vi "SIM Simulation init.vi"(0 "initial time":dbl format="%.2f", 1 "Nan/Inf Check":bool, 2 "continuous integrator":T3, 3 "Execution Mode":T1 items=["Simulate to Completion", "Single Time-Step Simulation (Fixed Step Only)"], 5 "final time":dbl=10.0 format="%.2f", 7 "time step":dbl=0.1 format="%.2f", 8 "error in (no error)":errorcluster, 9 "absolute tolerance":dbl=0.1 format="%.2e", 11 "relative tolerance":dbl=0.1 format="%.2e", 12 "maximum step size":dbl=0.1 format="%.2e", 13 "min step size":dbl=0.1, 14 "discrete time step":dbl=0.1, 15 "Simulation data":T2={"continuous integrator"=enum."RK 1 (Euler)", "initial time"=0.0, "final time"=0.0, "step size"=0.0, "proposed step size"=0.0, "max step size"=0.0, "min step size"=0.0, "discrete time step"=0.0, "max step ratio"=0.0, "Diag Eval Stage"=enum."Init", "Substep Index"=0, "Timestep Index"=0.0, "simulation time"=0.0, "current timestep base"=0.0, "proposed step time"=0.0, "absolute tolerance"=0.0, "relative tolerance"=0.0, "step accepted?"=TRUE, "step complete?"=FALSE, "Halt?"=FALSE, "reset integrator?"=FALSE, "machine epsilon"=0.0, "min float"=0.0, "error"={"status"=FALSE, "code"=0, "source"=""}, "Method Order"=0, "Finished Late [i-1]"=FALSE, "Discrete step?"=FALSE, "NaN and Inf check?"=FALSE, "Final Timestep Index"=0.0, "(maj+disc)or(init)?"=FALSE, "Full Solver Reset"=TRUE, "Execution Mode"=0, "check vector sizes?"=TRUE, "solver handles zc?"=FALSE, "Simulation Registry"={"Current Idx"=0, "Node Tags"=[], "Node Headers"=[], "Node Data"=[], "Cont State data"={"inputs"=[], "outputs"=[], "reset"=[], "lower limits"=[], "upper limits"=[], "limit types"=[], "reset types"=[], "initial conditions"=[], "reset I.C."=[], "limited?"=[], "State Names"=[]}, "DiscreteInfo"={"tick period (sec)"=0.0, "time (ticks)"=0, "fire?"=[], "registry"={"period (sec)"=[], "skew (sec)"=[], "period (tick)"=[], "skew (tick)"=[]}, "discrete \nblocks?"=FALSE, "steps per tick"=0.0, "steps to tick"=0.0, "discrete \ntick?"=FALSE}, "Disc State data"={"Disc States"=[], "State Names"=[]}, "Registry Error"={"Error Block ID"=0, "code"=0}, "ZC Indices"=[]}, "variable step solver?"=FALSE, "First Substep?"=FALSE, "Continuous States?"=FALSE} {"Execution Mode" items=["Simulate to Completion", "Single Time-Step Simulation (Fixed Step Only)"]; "min float" format="%.1e"; "proposed step size" format="%.1e"; "proposed step time" format="%.1e"; "max step ratio" format="%.1e"; "min step size" format="%.1e"; "machine epsilon" format="%.1e"; "discrete time step" format="%.1e"; "max step size" format="%.1e"; "current timestep base" format="%.1e"; "final time" format="%.1e"; "simulation time" format="%.1e"; "relative tolerance" format="%.1e"; "absolute tolerance" format="%.1e"; "Substep Index" format="%.1e"; "step size" format="%.1e"; "initial time" format="%.1e"}) -> (10 "Simulation data out":T2={"continuous integrator"=enum."RK 1 (Euler)", "initial time"=0.0, "final time"=0.0, "step size"=0.0, "proposed step size"=0.0, "max step size"=0.0, "min step size"=0.0, "discrete time step"=0.0, "max step ratio"=0.0, "Diag Eval Stage"=enum."Init", "Substep Index"=0, "Timestep Index"=0.0, "simulation time"=0.0, "current timestep base"=0.0, "proposed step time"=0.0, "absolute tolerance"=0.0, "relative tolerance"=0.0, "step accepted?"=TRUE, "step complete?"=FALSE, "Halt?"=FALSE, "reset integrator?"=FALSE, "machine epsilon"=0.0, "min float"=0.0, "error"={"status"=FALSE, "code"=0, "source"=""}, "Method Order"=0, "Finished Late [i-1]"=FALSE, "Discrete step?"=FALSE, "NaN and Inf check?"=FALSE, "Final Timestep Index"=0.0, "(maj+disc)or(init)?"=FALSE, "Full Solver Reset"=TRUE, "Execution Mode"=0, "check vector sizes?"=TRUE, "solver handles zc?"=FALSE, "Simulation Registry"={"Current Idx"=0, "Node Tags"=[], "Node Headers"=[], "Node Data"=[], "Cont State data"={"inputs"=[], "outputs"=[], "reset"=[], "lower limits"=[], "upper limits"=[], "limit types"=[], "reset types"=[], "initial conditions"=[], "reset I.C."=[], "limited?"=[], "State Names"=[]}, "DiscreteInfo"={"tick period (sec)"=0.0, "time (ticks)"=0, "fire?"=[], "registry"={"period (sec)"=[], "skew (sec)"=[], "period (tick)"=[], "skew (tick)"=[]}, "discrete \nblocks?"=FALSE, "steps per tick"=0.0, "steps to tick"=0.0, "discrete \ntick?"=FALSE}, "Disc State data"={"Disc States"=[], "State Names"=[]}, "Registry Error"={"Error Block ID"=0, "code"=0}, "ZC Indices"=[]}, "variable step solver?"=FALSE, "First Substep?"=FALSE, "Continuous States?"=FALSE} {"Execution Mode" items=["Simulate to Completion", "Single Time-Step Simulation (Fixed Step Only)"]; "min float" format="%.1e"; "proposed step size" format="%.1e"; "proposed step time" format="%.1e"; "max step ratio" format="%.1e"; "min step size" format="%.1e"; "machine epsilon" format="%.1e"; "discrete time step" format="%.1e"; "max step size" format="%.1e"; "current timestep base" format="%.1e"; "final time" format="%.1e"; "simulation time" format="%.1e"; "relative tolerance" format="%.1e"; "absolute tolerance" format="%.1e"; "Substep Index" format="%.1e"; "step size" format="%.1e"; "initial time" format="%.1e"})   [LabVIEW 2010]
uses:
  SIM simulation data.ctl
  SIM integration method.ctl
  SIM diagram eval stage.ctl
  SIMSCR Execution Mode.ctl
  SIM Simulation Registry.ctl
  SIM Registry Node Header.ctl
  SIM Registry Node Record.ctl
  SIM trigger type.ctl
  SIM solver state data.ctl
  SIM limit type.ctl
  SIM discrete data.ctl
  SIM Discrete state data.ctl
  SIM Simulation Registry Error.ctl
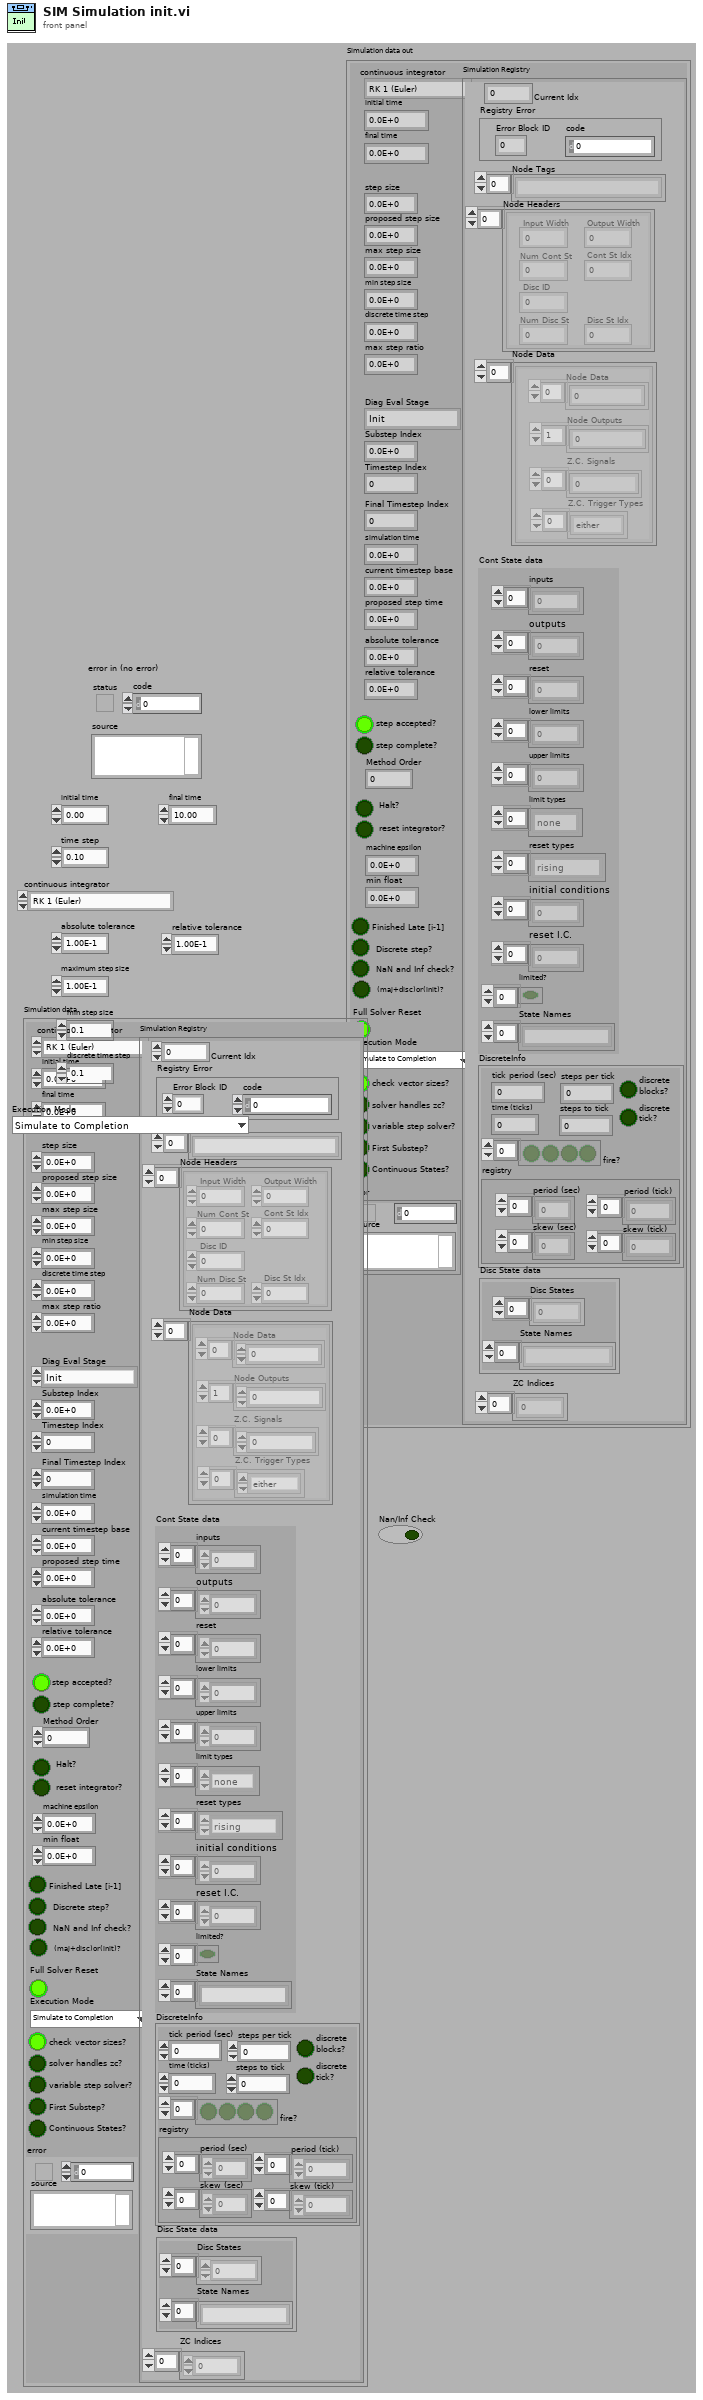
[diagram p1: front panel]
types:
  T1 = typedef "SIMSCR Execution Mode.ctl" = u16
  T2 = typedef "SIM simulation data.ctl" = cluster{"continuous integrator":T3, "initial time":dbl, "final time":dbl, "step size":dbl, "proposed step size":dbl, "max step size":dbl, "min step size":dbl, "discrete time step":dbl, "max step ratio":dbl, "Diag Eval Stage":T4, "Substep Index":i32, "Timestep Index":dbl, "simulation time":dbl, "current timestep base":dbl, "proposed step time":dbl, "absolute tolerance":dbl, "relative tolerance":dbl, "step accepted?":bool, "step complete?":bool, "Halt?":bool, "reset integrator?":bool, "machine epsilon":dbl, "min float":dbl, "error":errorcluster, "Method Order":u32, "Finished Late [i-1]":bool, "Discrete step?":bool, "NaN and Inf check?":bool, "Final Timestep Index":dbl, "(maj+disc)or(init)?":bool, "Full Solver Reset":bool, "Execution Mode":T1, "check vector sizes?":bool, "solver handles zc?":bool, "Simulation Registry":T5, "variable step solver?":bool, "First Substep?":bool, "Continuous States?":bool}
  T3 = typedef "SIM integration method.ctl" = enum16{"RK 1 (Euler)", "Linearizer", "State Query", "Trim Eval", "Adams", "RK 3", "RK 4", "RK 45", "BDF", "RK 2", "RK 23", "Rosenbrock", "Discrete States Only"}
  T4 = typedef "SIM diagram eval stage.ctl" = enum16{"Init", "Minor Substep", "Major Substep", "Final"}
  T5 = typedef "SIM Simulation Registry.ctl" = cluster{"Current Idx":i32, "Node Tags":string[], "Node Headers":T6[], "Node Data":T7[], "Cont State data":T9, "DiscreteInfo":T11, "Disc State data":T12, "Registry Error":T13, "ZC Indices":i32[]}
  T6 = typedef "SIM Registry Node Header.ctl" = cluster{"Input Width":i32, "Disc ID":i32, "Num Cont St":i32, "Cont St Idx":i32, "Num Disc St":i32, "Disc St Idx":i32, "Output Width":i32}
  T7 = typedef "SIM Registry Node Record.ctl" = cluster{"Node Data":dbl[], "Node Outputs":dbl[], "Z.C. Signals":dbl[], "Z.C. Trigger Types":T8[]}
  T8 = typedef "SIM trigger type.ctl" = enum16{"rising", "falling", "either", "none"}
  T9 = typedef "SIM solver state data.ctl" = cluster{"inputs":dbl[], "outputs":dbl[], "reset":dbl[], "lower limits":dbl[], "upper limits":dbl[], "limit types":T10[], "reset types":T8[], "initial conditions":dbl[], "reset I.C.":dbl[], "limited?":bool[], "State Names":string[]}
  T10 = typedef "SIM limit type.ctl" = enum16{"upper", "lower", "both", "none"}
  T11 = typedef "SIM discrete data.ctl" = cluster{"tick period (sec)":dbl, "time (ticks)":i32, "fire?":bool[], "registry":cluster{"period (sec)":dbl[], "skew (sec)":dbl[], "period (tick)":i32[], "skew (tick)":i32[]}, "discrete \nblocks?":bool, "steps per tick":dbl, "steps to tick":dbl, "discrete \ntick?":bool}
  T12 = typedef "SIM Discrete state data.ctl" = cluster{"Disc States":dbl[], "State Names":string[]}
  T13 = typedef "SIM Simulation Registry Error.ctl" = cluster{"Error Block ID":i32, "code":i32}
  T14 = enum16{"Fixed Step-Size Solver", "Variable Step-Size Solver"}
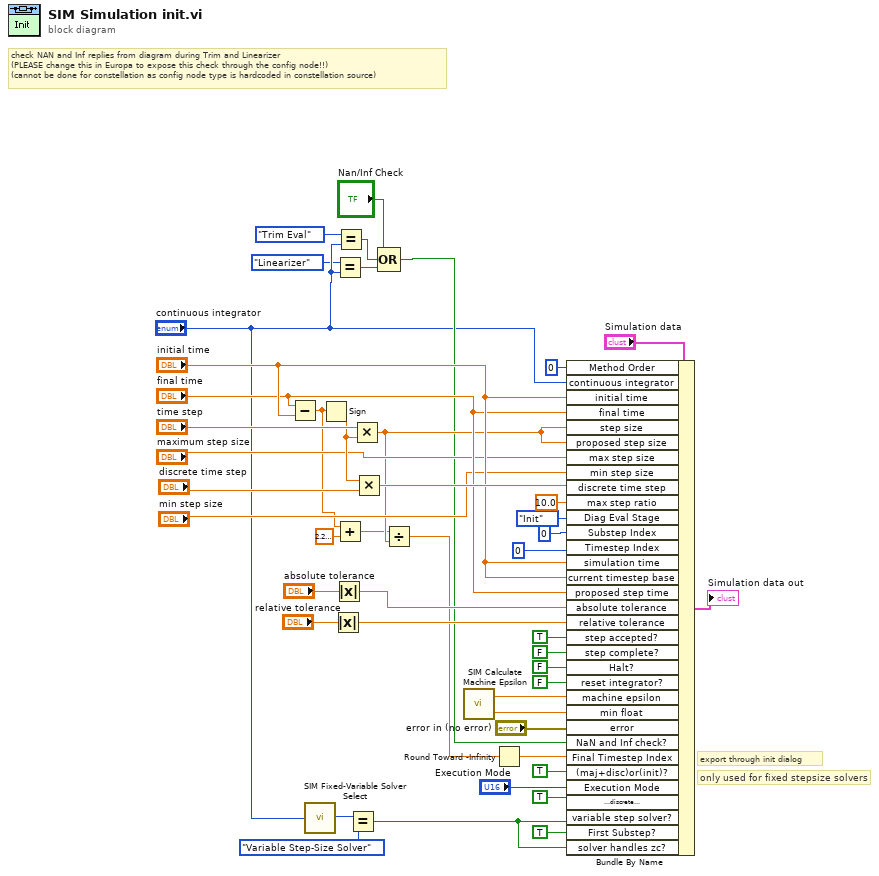
[diagram p0: block diagram]
diagram:
  # "check NAN and Inf replies from diagram during Trim and Linearizer\n(PLEASE change this in Europa to expose this check through the config node!!)\n(cannot be done for constellation as config node type is hardcoded in constellation source)"
  # "only used for fixed stepsize solvers"
  # "export through init dialog"
  n1 = Subtract(x="final time", y="initial time") -> (x-y=w21:dbl)
  n2 = call "SIM Fixed-Variable Solver Select.vi"("continuous integrator"="continuous integrator") -> ("Solver Type"=w9:T14)
  n3 = Sign(1:w21) -> (0:w26:dbl)
  n4 = Absolute Value(x="relative tolerance") -> (abs(x)=w31:dbl)
  n5 = Absolute Value(x="absolute tolerance") -> (abs(x)=w32:dbl)
  n6 = Equal?(x=SIM_integration_method."Linearizer", y="continuous integrator") -> (x = y?=w4:bool)
  n7 = Add(x=w21, y=2.220446049250313e-16) -> (x+y=w15:dbl)
  n8 = Equal?(x=SIM_integration_method."Trim Eval", y="continuous integrator") -> (x = y?=w5:bool)
  n9 = Equal?(x=w9, y=T14."Variable Step-Size Solver") -> (x = y?=w6:bool)
  n10 = Multiply(x="time step", y=w26) -> (x*y=w20:dbl)
  n11 = Multiply(x=w26, y="discrete time step") -> (x*y=w27:dbl)
  n12 = Compound Arithmetic op=OR("Nan/Inf Check", w5, w4) -> (w12:bool)
  n13 = Divide(x=w15, y=w20) -> (x/y=w16:dbl)
  n14 = call "SIM Calculate Machine Epsilon.vi"() -> ("min float"=w33:dbl, "machine eps"=w34:dbl)
  n15 = Round Toward -Infinity(1:w16) -> (0:w11:dbl)
  n16 = Bundle By Name(cluster="Simulation data", "Method Order"=u32 0, "continuous integrator"="continuous integrator", "initial time"="initial time", "final time"="final time", "step size"=w20, "proposed step size"=w20, "max step size"="maximum step size", "min step size"="min step size", "discrete time step"=w27, "max step ratio"=10.0, "Diag Eval Stage"=SIM_diagram_eval_stage."Init", "Substep Index"=0, "Timestep Index"=u64 0, "simulation time"="initial time", "current timestep base"="initial time", "proposed step time"="final time", "absolute tolerance"=w32, "relative tolerance"=w31, "step accepted?"=TRUE, "step complete?"=FALSE, "Halt?"=FALSE, "reset integrator?"=FALSE, "machine epsilon"=w34, "min float"=w33, "error"="error in (no error)", "NaN and Inf check?"=w12, "Final Timestep Index"=w11, "(maj+disc)or(init)?"=TRUE, "Execution Mode"="Execution Mode", "Simulation Registry.DiscreteInfo.discrete \ntick?"=TRUE ("DiscreteInfo.discrete \ntick?"), "variable step solver?"=w6, "First Substep?"=TRUE, "solver handles zc?"=w6) -> (→"Simulation data out":T2)
